vi "Set Active Point.vi"(0 "eye scan single point":refnum<class "niHighSpeedSerial Eye Scan Single Point v1 Host.lvclass">, 5 "active point":T1, 11 "error in":errorcluster) -> (4 "eye scan single point out":refnum<class "niHighSpeedSerial Eye Scan Single Point v1 Host.lvclass">, 15 "error out":errorcluster)   [LabVIEW 2014, in "niHighSpeedSerial Eye Scan Single Point v1 Host.lvclass"]
doc: "Configures the hardware with the point to measure (vertical and horizontal offsets).\n\n<B>Input Parameters</B>\n\n<B>eye scan single point</B> takes in a reference to your session from the previous VI.\n\n<B>active point</B> is the point to measure\n\n<B>active point.horizontal offset</B> is the horizontal offset of the point to measure.\n\n<B>active point.vertical offset</B> is the vertical offset of the point to measure.\n\n<B>error in</B> describes error conditions that occur before this node runs. This input provides standard 'error in' functionality.\n\n<B>Output Parameters</B>\n\n<B>eye scan single point out</B> passes a reference to your session to the next VI.\n\n<B>error out</B> contains error information. This output provides standard 'error out' functionality."
uses:
  <instrlib>/niHighSpeedSerial/Eye Scan/v1/Host/Impl/Single Point/niHighSpeedSerial Eye Scan Single Point v1 Host.lvclass
  <instrlib>/niHighSpeedSerial/Eye Scan/v1/Host/Common/Public/Point Offsets.ctl
  <instrlib>/niHighSpeedSerial/Eye Scan/v1/Host/Impl/Single Point/niHighSpeedSerial Eye Scan Single Point v1 Host.lvclass/niHighSpeedSerial Eye Scan Single Point v1 Host.ctl
  <instrlib>/niHighSpeedSerial/Eye Scan/v1/Host/Impl/Single Point/Private/Channel Measure State.ctl
  <instrlib>/niHighSpeedSerial/Eye Scan/v1/Host/Common/niHighSpeedSerial Eye Scan Common v1 Host.lvlib
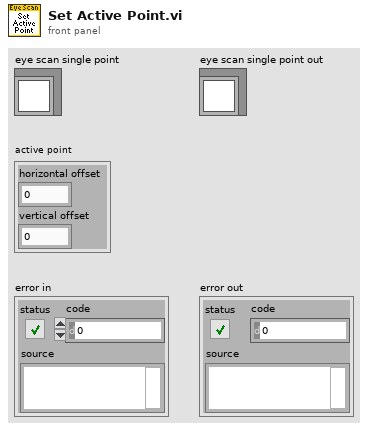
[diagram p1: front panel]
types:
  T1 = typedef "niHighSpeedSerial Eye Scan Common v1 Host.lvlib/Point Offsets.ctl" = cluster{"horizontal offset":i16, "vertical offset":i8}
  T2 = typedef "niHighSpeedSerial Eye Scan Single Point v1 Host.lvclass/Channel Measure State.ctl" = enum16{"Uninitialized", "Initialized", "Ready", "Request", "Wait", "Read", "Process", "Finished"}
  T3 = typedef "niHighSpeedSerial Eye Scan Single Point v1 Host.lvclass/Private Data.ctl" = cluster{"GTX2_CHANNEL register map":refnum<class "GTX2_CHANNEL Register Map.lvclass">, "instruction target":refnum<class "niInstr Instruction Target v1 Host.lvclass">, "channel measure state":T2, "in DFE mode?":bool, "prescale":u8, "receiver data width":T4, "active point":T1, "ut sign":T5, "positive counts":T6, "negative counts":T6}
  T4 = typedef "niHighSpeedSerial Eye Scan Common v1 Host.lvlib/Data Width.ctl" = enum16{"16 Bit", "20 Bit", "32 Bit", "40 Bit"}
  T5 = typedef "GTX2_CHANNEL v1 Host.lvlib/ESVertOffsetSign.ctl" = enum8{"Positive", "Negative"}
  T6 = typedef "niHighSpeedSerial Eye Scan Single Point v1 Host.lvclass/Counts.ctl" = cluster{"sample count":u64, "error count":u16}
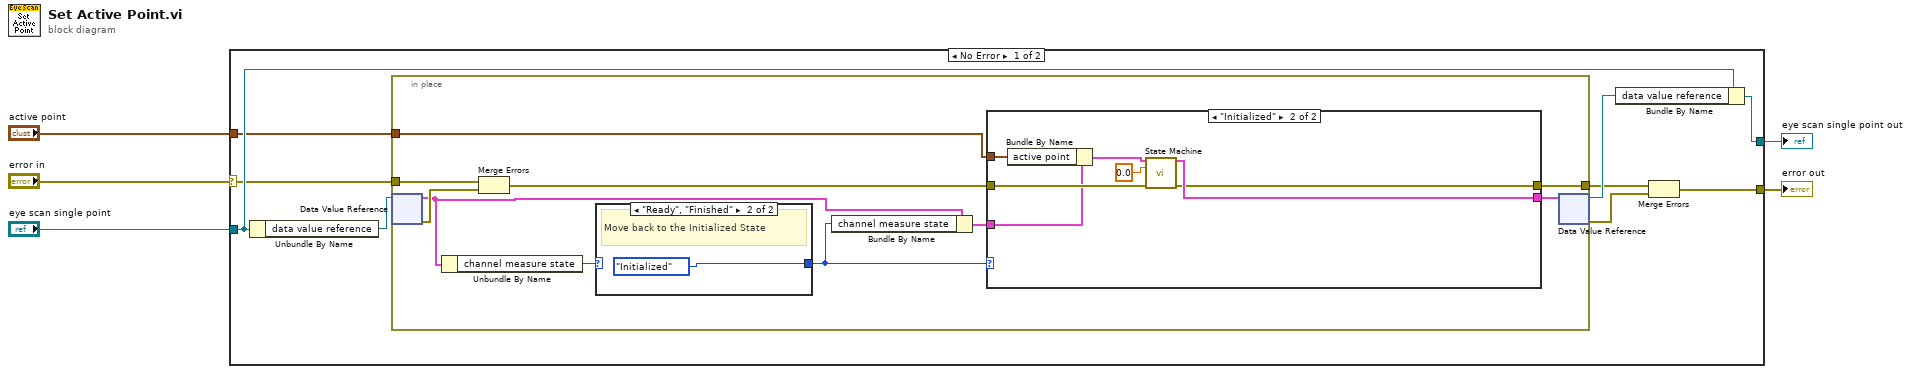
[diagram p0: block diagram]
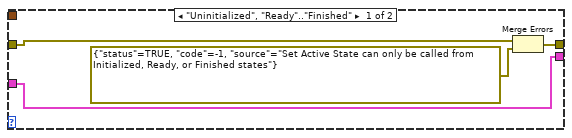
[diagram p3: hidden frame]
diagram:
  n1 = case shown="No Error" "error in" {
    selector: "error in" -> [w11 w39]
    tunnel: [w8 w39] -> w4
    tunnel: [w7 w38] -> w3
    tunnel: "eye scan single point" -> [w13 w38]
    tunnel: "active point" -> [w6 _]
    frame No Error {
      n2 = Unbundle By Name(w13) -> ("data value reference"=w14:refnum<data-value>)
      n3 = in-place {
        in-place-border: w11 -> [w24]
        in-place-border: [w20] -> w10
        in-place-border: w6 -> [w15]
        n4 = in-place-dvr #1(w14) -> (w19:T3, w23:errorcluster)
        n5 = Unbundle By Name(w19) -> ("channel measure state"=w17:T2)
        n6 = Merge Errors(w24, w23) -> (w21:errorcluster)
        n7 = case shown="\"Ready\", \"Finished\"" w17 {
          selector: w17 -> [w25 _]
          tunnel: [w25 Channel_Measure_State."Initialized" ("t")] -> w16
          frame "Uninitialized", "Initialized", "Request".."Process" {
          }
          frame "Ready", "Finished" {
            # "Move back to the Initialized State"
          }
        }
        n8 = Bundle By Name(cluster=w19, "channel measure state"=w16) -> (w18:T3)
        n9 = case shown="\"Initialized\"" w16 {
          tunnel: [w27 w36] -> w22
          tunnel: w21 -> [w30 w34]
          tunnel: [w28 w33] -> w20
          tunnel: w18 -> [w27 w32]
          tunnel: w15 -> [_ w31]
          frame "Uninitialized", "Ready".."Finished" {
            n10 = Merge Errors(w30, errorcluster {"status"=TRUE, "code"=-1, "source"="Set Active State can only be called from Initialized, Ready, or Finished states"} ("error IO")) -> (w28:errorcluster)
          }
          frame "Initialized" {
            n11 = Bundle By Name(cluster=w32, "active point"=w31) -> (w37:T3)
            n12 = call <instrlib>:"State Machine.vi"("private data"=w37, "timeout (100 ms)"=0.0 ("Timeout (100 ms)"), "error in"=w34) -> ("private data out"=w36:T3, "error out"=w33:errorcluster)  [unwired: 6 in, 5 out]
          }
        }
        n13 = in-place-dvr #1(w22) -> (w12:refnum<data-value>, w9:errorcluster)
      }
      n14 = Bundle By Name(cluster=w13, "data value reference"=w12) -> (w7:refnum<class "niHighSpeedSerial Eye Scan Single Point v1 Host.lvclass">)
      n15 = Merge Errors(w10, w9) -> (w8:errorcluster)
    }
    frame Error {
    }
  }
  "error out" <- w4
  "eye scan single point out" <- w3
